vi "Main.vi"() -> ()   [LabVIEW 2024]
doc: "This template is for the Queued Message Handler design pattern.\n\nThe Event Handling Loop generates messages based on user interface actions.\n\nThe Message Handling Loop processes messages generated by the Event Handling Loop, or by other messages. The messages are string values, so new messages can be added easily to the Message Cases case structure in the Message Handling Loop. Each message cluster can also provide an optional value for Message Data, which is a variant that can be converted to whatever message-specific data is required."
uses:
  controls/UI Data.ctl
  controls/self.ctl
  controls/channelDefinition.ctl
  support/Message Queue/Enqueue Message (Single).vi
  <vilib>/Utility/error.llb/Error Cluster From Error Code.vi
  <vilib>/ErrorRing/Error Ring.xnode
  support/Message Queue/Message Queue.lvlib
  support/User Event - Stop/User Event - Stop.lvlib
panel:
  in  "configPath":path=path "C:/Users/miles/OneDrive - Embry-Riddle Aeronautical University/Admin/Facilities/TC3/TC3 DAC/Code/Sandbox/Node based/controlNode/Configuration/nodeConfig_0.xlsx"
  out "Status":string
  in  "Restart Connections":bool
  in  "Exit":bool
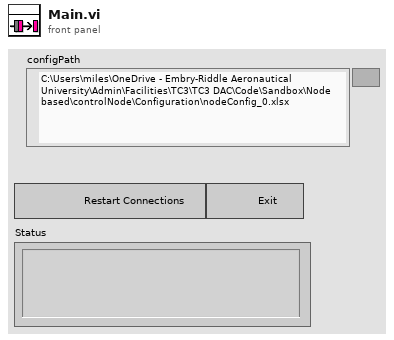
[diagram p1: front panel]
types:
  T1 = typedef "self.ctl" = cluster{"refDes":string, "IP":string, "DI":i32, "DO":i32, "AI":i32, "AO":i32, "Description":string, "TC":i32, "channelDefinitions":T2[]}
  T2 = typedef "channelDefinition.ctl" = cluster{"channel":string, "refDes":string, "units":string, "slope":dbl, "offset":dbl, "type":string}
  T3 = typedef "UI Data.ctl" = cluster{"Node Enable":bool, "Node Ref":string, "Numeric <Replace Me>":dbl, "Restart Connections Ref":refnum<vi>, "Status Display Ref":refnum<vi>, "Exit Button Ref":refnum<vi>}
  T4 = typedef "Message Queue.lvlib/All Message Queues.ctl" = cluster{"UI":refnum<queue>, "daqStreams":refnum<queue>, "userStreams":refnum<queue>, "logging":refnum<queue>}
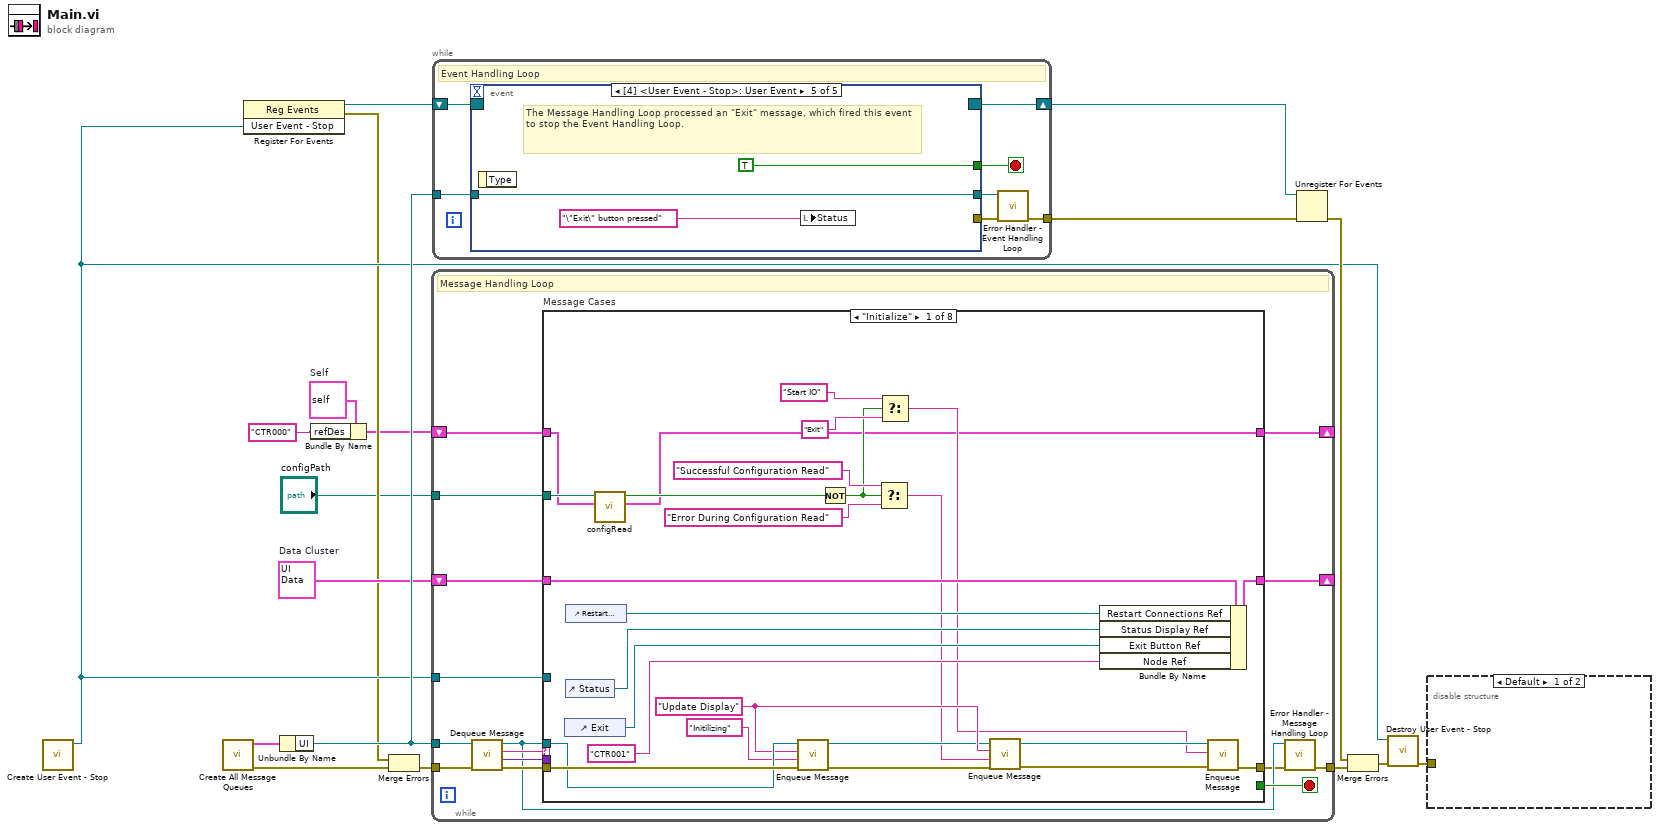
[diagram p0: block diagram]
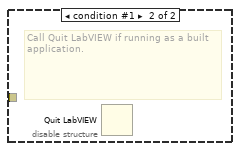
[diagram p2: hidden frame]
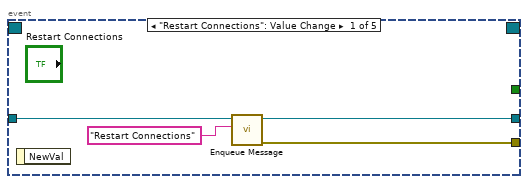
[diagram p3: hidden frame]
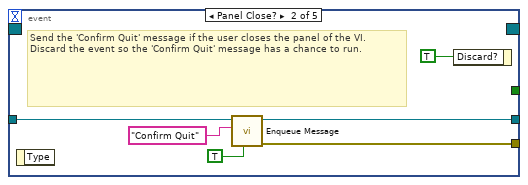
[diagram p4: hidden frame]
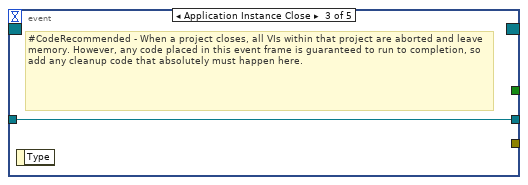
[diagram p5: hidden frame]
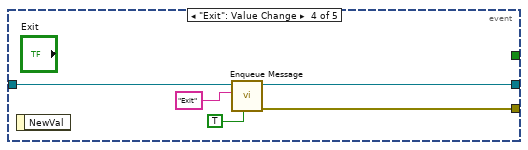
[diagram p6: hidden frame]
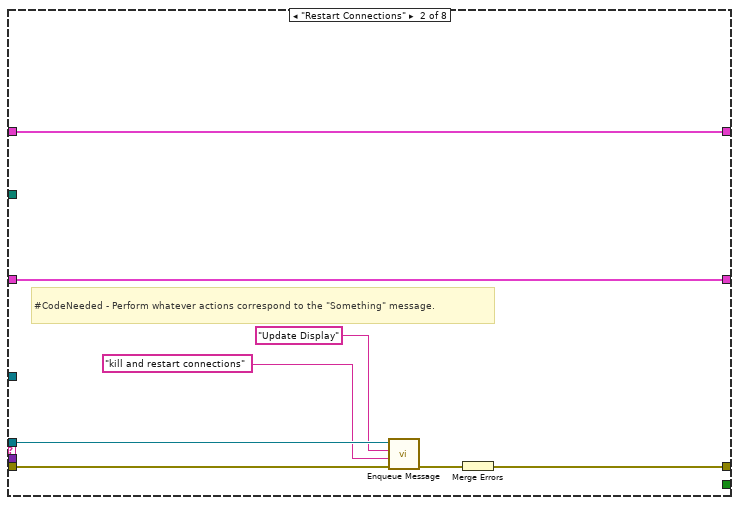
[diagram p7: hidden frame]
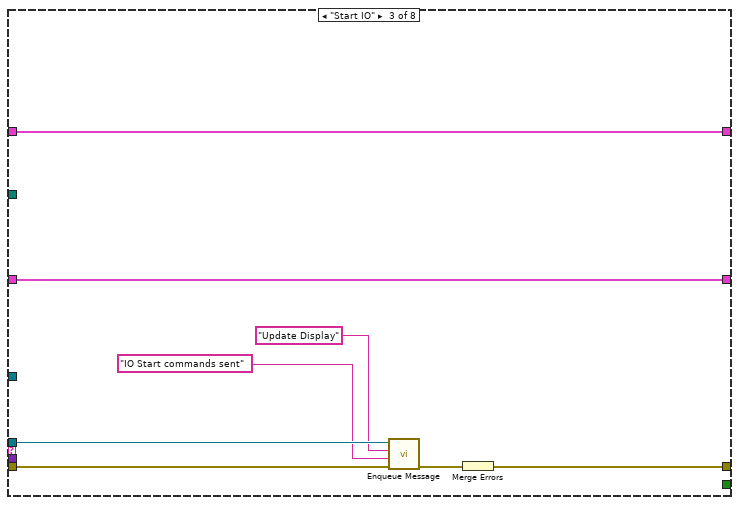
[diagram p8: hidden frame]
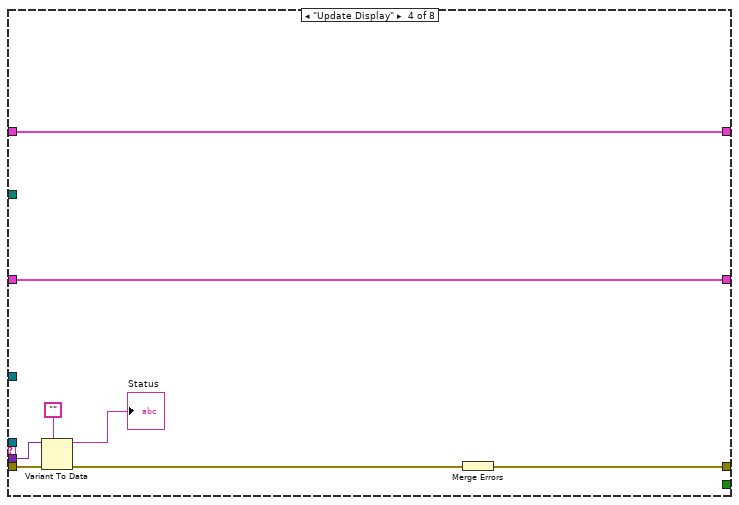
[diagram p9: hidden frame]
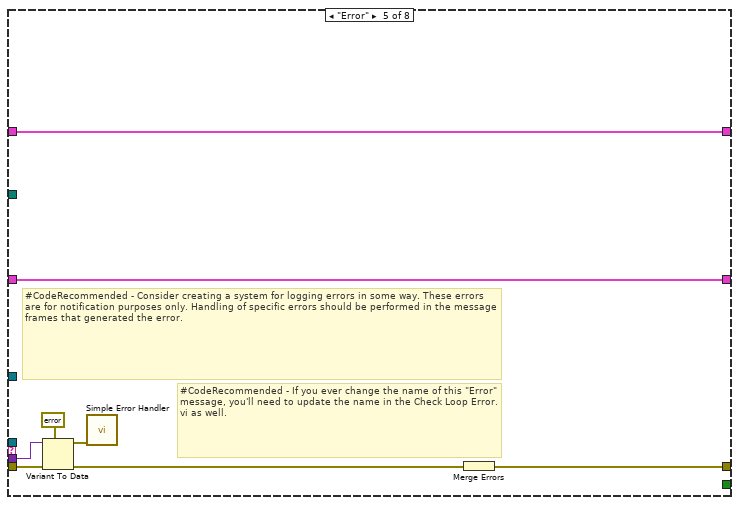
[diagram p10: hidden frame]
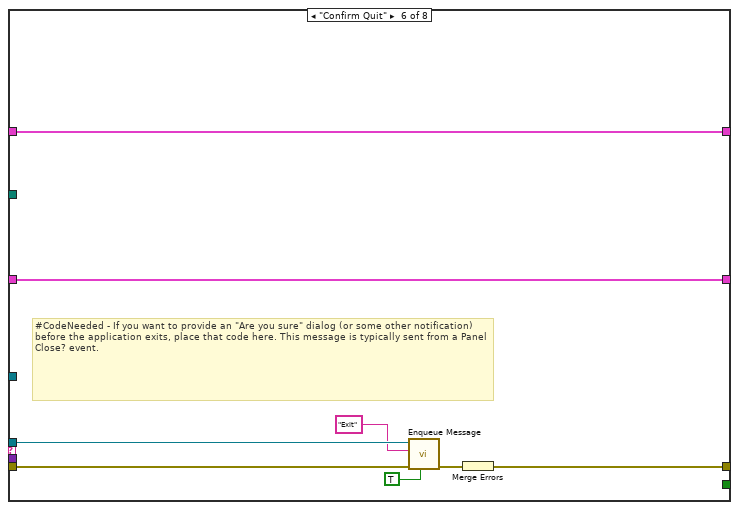
[diagram p11: hidden frame]
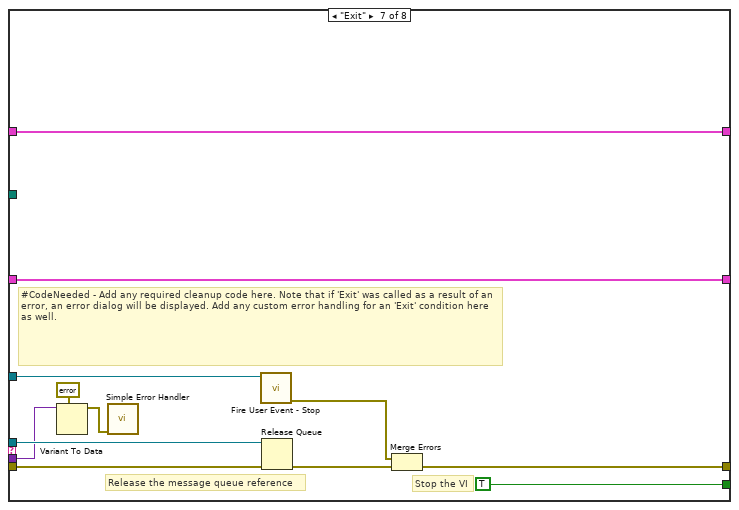
[diagram p12: hidden frame]
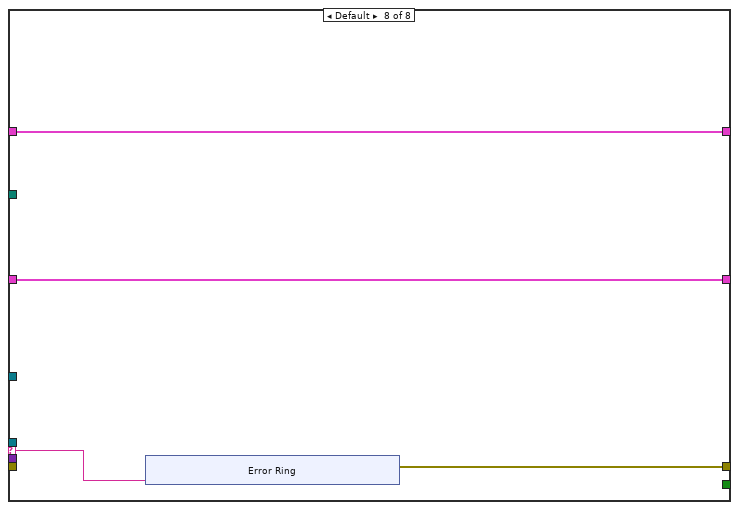
[diagram p13: hidden frame]
diagram:
  w3 = T1 {"refDes"="ERR000", "IP"="localhost", "DI"=0, "DO"=0, "AI"=0, "AO"=0, "Description"="ERR", "TC"=0, "channelDefinitions"=[]}  # Self
  w11 = T3 {"Node Enable"=FALSE, "Node Ref"="", "Numeric <Replace Me>"=0.0, "Restart Connections Ref"=refnum, "Status Display Ref"=refnum, "Exit Button Ref"=refnum}  # Data Cluster
  n1 = call "Create User Event - Stop.vi"() -> ("User Event - Stop"=w7:refnum<user-event>)  [unwired: 10 in, 1 out]
  n2 = call "Create All Message Queues.vi"() -> ("error out"=w18:errorcluster, "Message Queues out"=w17:T4)  [unwired: 10 in]
  n3 = register-events(w7) -> (reference out=w8:refnum<event-registration>, error out=w5:errorcluster)  [unwired: 2 in]
  n4 = Unbundle By Name(w17) -> ("UI"=w15:refnum<queue>)
  n5 = Bundle By Name(cluster=w3, "refDes"="CTR000") -> (w2:T1)
  n6 = Merge Errors(w5, w18) -> (w6:errorcluster)
  n7 = while {
    tunnel: w15 -> [w25]
    shift-right: [w32] -> _
    shift-left: w11 -> [w33]
    tunnel: w7 -> [w30]
    tunnel: w6 -> [w29]
    tunnel: [w23] -> w16
    tunnel: "configPath" -> [w21]
    shift-right: [w20] -> _
    shift-left: w2 -> [w19]
    stop <- w31 stop-if-true
    # "Message Handling Loop"
    n8 = call "Dequeue Message.vi"("error in (no error)"=w29, "Message Queue"=w25) -> ("error out"=w28:errorcluster, "Message Data"=w26:variant, "Message"=w27:string, "dup Message Queue"=w24:refnum<queue>)  [unwired: 6 in]
    n9 = case "Message Cases" shown="\"Initialize\"" w27 {
      selector: w27 -> [_ _ _ _ _ _ _ w113]
      tunnel: w24 -> [w54 w63 w71 _ _ w95 w111 _]
      tunnel: w28 -> [w59 w65 w73 w81 w91 w99 w104 _]
      tunnel: [w50 w66 w74 w82 w85 w97 w107 w114] -> w22
      tunnel: w33 -> [w58 w67 w75 w83 w90 w98 w110 w115]
      tunnel: [w57 w67 w75 w83 w90 w98 w110 w115] -> w32
      tunnel: [_ _ _ _ _ _ TRUE _] -> w31
      tunnel: w26 -> [_ _ _ w80 w89 _ w101 _]
      tunnel: w30 -> [_ _ _ _ _ _ w106 _]
      tunnel: w21 -> [w49 _ _ _ _ _ _ _]
      tunnel: [w34 w60 w68 w76 w84 w92 w100 w112] -> w20
      tunnel: w19 -> [w35 w60 w68 w76 w84 w92 w100 w112]
      frame "Initialize" {
        w48 = "Update Display" ("Message")
        # "Initialize - All initialization work should take place in this message, since other loops can potentially enqueue messages that execute immediately after this one."
        n10 = control-ref of="Exit"() -> (w55:refnum<vi>)
        n11 = control-ref of="Restart Connections"() -> (w52:refnum<vi>)
        n12 = control-ref of="Status"() -> (w56:refnum<vi>)
        n13 = call "configRead.vi"("Self"=w35, "configPath"=w49) -> ("Self"=w34:T1, "Cancel/Err"=w41:bool)  [unwired: 8 in]
        n14 = call-poly "Enqueue Message.vi"("error in (no error)"=w59, "Message Data"="Initilizing", "Message"=w48, "Message Queue"=w54) -> ("error out"=w46:errorcluster, "dup Message Queue"=w47:refnum<queue>)  [unwired: 6 in]
        n15 = Not(x=w41) -> (.not. x?=w36:bool)
        n16 = Select(t="Successful Configuration Read", s=w36, f="Error During Configuration Read") -> (s? t:f=w43:string)
        n17 = Select(t="Start IO" ("Message"), s=w36, f="Exit" ("Message")) -> (s? t:f=w42:string)
        n18 = call-poly "Enqueue Message.vi"("error in (no error)"=w46, "Message Data"=w43, "Message"=w48, "Message Queue"=w47) -> ("error out"=w45:errorcluster, "dup Message Queue"=w44:refnum<queue>)  [unwired: 6 in]
        n19 = Bundle By Name(cluster=w58, "Restart Connections Ref"=w52, "Status Display Ref"=w56, "Exit Button Ref"=w55, "Node Ref"="CTR001" ("Initial Message")) -> (w57:T3)
        n20 = call-poly "Enqueue Message.vi"("error in (no error)"=w45, "Message"=w42, "Message Queue"=w44) -> ("error out"=w50:errorcluster)  [unwired: 7 in, 1 out]
      }
      frame "Restart Connections" {
        # "#CodeNeeded - Perform whatever actions correspond to the \"Something\" message."
        # "Something - Replace this message with functionality for your own application."
        n21 = call-poly "Enqueue Message.vi"("error in (no error)"=w65, "Message Data"="kill and restart connections" ("\"Do Something\" button pressed"), "Message"="Update Display", "Message Queue"=w63) -> ("error out"=w64:errorcluster)  [unwired: 6 in, 1 out]
        n22 = Merge Errors(w64) -> (w66:errorcluster)
      }
      frame "Start IO" {
        # "Something - Replace this message with functionality for your own application."
        n23 = call-poly "Enqueue Message.vi"("error in (no error)"=w73, "Message Data"="IO Start commands sent" ("\"Do Something\" button pressed"), "Message"="Update Display", "Message Queue"=w71) -> ("error out"=w72:errorcluster)  [unwired: 6 in, 1 out]
        n24 = Merge Errors(w72) -> (w74:errorcluster)
      }
      frame "Update Display" {
        # "Update Display - Convert the message data to a string to display in the Data Display indicator."
        n25 = Variant To Data(error in=w81, type="", Variant=w80) -> (data=→"Status":string, error out=w78:errorcluster)
        n26 = Merge Errors(w78) -> (w82:errorcluster)
      }
      frame "Error" {
        # "#CodeRecommended - If you ever change the name of this \"Error\" message, you'll need to update the name in the Check Loop Error.vi as well."
        # "#CodeRecommended - Consider creating a system for logging errors in some way. These errors are for notification purposes only. Handling of specific errors should be performed in the message frames that generated the error."
        # "Error - Display an error dialog. This message is sent by the \"Error Handler\" VIs at the end of other loops in this application."
        n27 = Variant To Data(error in=w91, type=errorcluster {"status"=FALSE, "code"=0, "source"=""} ("error constant"), Variant=w89) -> (data=w87:errorcluster, error out=w86:errorcluster)
        n28 = call <vilib>:"Simple Error Handler.vi"("error in (no error)"=w87) -> ()  [unwired: 4 in, 5 out]
        n29 = Merge Errors(w86) -> (w85:errorcluster)
      }
      frame "Confirm Quit" {
        # "#CodeNeeded - If you want to provide an \"Are you sure\" dialog (or some other notification) before the application exits, place that code here. This message is typically sent from a Panel Close? event."
        # "Confirm Quit - Message that can confirm whether or not the user wants to exit the application."
        n30 = call-poly "Enqueue Message.vi"("Priority Message? (F)"=TRUE, "error in (no error)"=w99, "Message"="Exit", "Message Queue"=w95) -> ("error out"=w96:errorcluster)  [unwired: 6 in, 1 out]
        n31 = Merge Errors(w96) -> (w97:errorcluster)
      }
      frame "Exit" {
        # "Stop the VI"
        # "Release the message queue reference"
        # "#CodeNeeded - Add any required cleanup code here. Note that if 'Exit' was called as a result of an error, an error dialog will be displayed. Add any custom error handling for an 'Exit' condition here as well."
        # "Exit - Exit the application."
        n32 = Variant To Data(type=errorcluster {"status"=FALSE, "code"=0, "source"=""} ("error constant"), Variant=w101) -> (data=w102:errorcluster)  [unwired: 1 in, 1 out]
        n33 = call <vilib>:"Simple Error Handler.vi"("error in (no error)"=w102) -> ()  [unwired: 4 in, 5 out]
        n34 = call "Fire User Event - Stop.vi"("User Event - Stop"=w106) -> ("error out"=w105:errorcluster)  [unwired: 10 in]
        n35 = Release Queue(queue=w111, error in (no error)=w104) -> (error out=w108:errorcluster)  [unwired: 1 in, 2 out]
        n36 = Merge Errors(w105, w108) -> (w107:errorcluster)
      }
      frame Default {
        # "'Default' case only runs if there is a message that isn't defined in any of the other cases.  Output a programming error."
        n37 = xnode "Error Ring"("parameter 0"=w113) -> ("error out"=w114:errorcluster)
      }
    }
    n38 = call "Error Handler - Message Handling Loop.vi"("error in (no error)"=w22, "Message Queue"=w24) -> ("dup error in"=w23:errorcluster)  [unwired: 8 in, 1 out]
  }
  n39 = while {
    tunnel: w15 -> [w129]
    shift-right: [w127] -> w12
    shift-left: w8 -> [w128]
    tunnel: [w123] -> w9
    stop <- w125 stop-if-true
    # "Event Handling Loop"
    n40 = event shown="[4] <User Event - Stop>: User Event" {
      selector: w128 -> [_ _ _ _ _]
      dyn-events: [_ _ _ _ _] -> w127
      timeout: _ -> [_ _ _ _ _]
      tunnel: [_ _ _ _ TRUE ("Discard?")] -> w125
      tunnel: w129 -> [w133 w138 w140 w145 w148]
      tunnel: [w130 w137 _ w144 _] -> w126
      tunnel: [w132 w136 w140 w143 w148] -> w124
      event "Restart Connections": Value Change {
        n41 = event-data() -> ()  [unwired: 1 in, 1 out]
        n42 = call-poly "Enqueue Message.vi"("Message"="Restart Connections", "Message Queue"=w133) -> ("error out"=w130:errorcluster, "dup Message Queue"=w132:refnum<queue>)  [unwired: 8 in]
      }
      event Panel Close? {
        # "Send the 'Confirm Quit' message if the user closes the panel of the VI. Discard the event so the 'Confirm Quit' message has a chance to run."
        n43 = event-data() -> ()  [unwired: 1 in, 1 out]
        n44 = call-poly "Enqueue Message.vi"("Priority Message? (F)"=TRUE, "Message"="Confirm Quit", "Message Queue"=w138) -> ("error out"=w137:errorcluster, "dup Message Queue"=w136:refnum<queue>)  [unwired: 7 in]
        n45 = event-data("Discard?"=TRUE) -> ()  [unwired: 1 in, 1 out]
      }
      event Application Instance Close {
        # "#CodeRecommended - When a project closes, all VIs within that project are aborted and leave memory. However, any code placed in this event frame is guaranteed to run to completion, so add any cleanup code that absolutely must happen here."
        n46 = event-data() -> ()  [unwired: 1 in, 1 out]
      }
      event "Exit": Value Change {
        n47 = event-data() -> ()  [unwired: 1 in, 1 out]
        n48 = call-poly "Enqueue Message.vi"("Priority Message? (F)"=TRUE, "Message"="Exit", "Message Queue"=w145) -> ("error out"=w144:errorcluster, "dup Message Queue"=w143:refnum<queue>)  [unwired: 7 in]
      }
      event User Event {
        # "The Message Handling Loop processed an \"Exit\" message, which fired this event to stop the Event Handling Loop."
        n49 = event-data() -> ()  [unwired: 1 in, 1 out]
        n50 = local write "Status"("\"Exit\" button pressed" ("VI Stopped")) -> ()
      }
    }
    n51 = call "Error Handler - Event Handling Loop.vi"("error in (no error)"=w126, "Message Queue"=w124) -> ("dup error in"=w123:errorcluster)  [unwired: 8 in, 1 out]
  }
  n52 = Unregister For Events(event registration refnum=w12, error in=w9) -> (error out=w13:errorcluster)
  n53 = Merge Errors(w13, w16) -> (w14:errorcluster)
  n54 = call "Destroy User Event - Stop.vi"("error in (no error)"=w14, "User Event - Stop"=w7) -> ("error out"=w10:errorcluster)  [unwired: 9 in]
  n55 = disable-structure shown="Default" {
    disable-tunnel: w10 -> [_ _]
    frame condition #0 (active) {
    }
    frame condition #1 {
      # "Call Quit LabVIEW if running as a built application."
      n56 = Quit LabVIEW() -> ()  [unwired: 1 in]
    }
  }
